vi "PWM Simulation.vi"() -> ()   [LabVIEW 2019]
uses:
  <vilib>/Simulation/Scripting/Companion Diagram/SimConfigNode/SimParams.ctl
  <vilib>/Simulation/Scripting/Companion Diagram/SimConfigNode/_simSolvers.ctl
  <vilib>/Simulation/Implementation/Shared/SIMSCR Execution Mode.ctl
  <vilib>/Platform/TimedLoop/XDataNode/timing_clust.ctl
  <vilib>/Platform/TimedLoop/XDataNode/nitl_modes.ctl
  <vilib>/Platform/TimedLoop/XDataNode/wakeup.ctl
  <vilib>/Simulation/Param Hierarchy/Typedefs/SIMPH Param Control Actions.ctl
  <vilib>/Simulation/Implementation/Shared/NILVSim_ParamChanged.vi
  <vilib>/Simulation/Implementation/Shared/NILVSim_FinishedLate.vi
  <vilib>/Simulation/Implementation/Shared/NILVSIM_BeginStep.vi
  <vilib>/Simulation/SignalDisplay/Implementation/NILVSim Time Waveform.llb/SIM Time Waveform (scalar).vi
  <vilib>/Simulation/Utility/Implementation/SIM Halt.vi
  <vilib>/Simulation/Implementation/Shared/NILVSim_Manager.vi
  <vilib>/Utility/error.llb/Clear Errors.vi
  <vilib>/Simulation/Implementation/Shared/NILVSim_FinalizeModel.vi
  <vilib>/Simulation/Implementation/Shared/SIM Unbundle Sim Info.vi
  <vilib>/Simulation/Implementation/Shared/SIMSH Read Queue.vi
  <vilib>/Simulation/Implementation/Shared/NILVSim_Initialize.vi
  Pulse Generator.vi
  <vilib>/Simulation/Utility/Implementation/NILVSim Get Time and IsAcceptedStep.vi
  <vilib>/Simulation/Implementation/Shared/NILVSim_GetModelError.vi
  <vilib>/Simulation/Implementation/Shared/SIM Bundle Sim Info.vi
  <vilib>/Simulation/Scripting/Companion Diagram/SimConfigNode/SimDog.xnode
  <vilib>/Platform/TimedLoop/XDataNode/XDataNode.xnode
  <vilib>/Simulation/Implementation/XNodeFramework/SimXNode/SimX.xnode
  <vilib>/Platform/TimedLoop/XDataNode/XDNodeRunTimeDep.lvlib
  <vilib>/Simulation/Implementation/Shared/NI_SIM_Implementation.lvlib
panel:
  in  "Stop Button":bool
  out "Threshold":dbl=50.0
  in  "Frequency (Hz)":dbl=1.0 min=0.0 max=10.0 step=0.01
  out "Boolean Pulse":waveform(dbl)(graph)={"t0"=timestamp(12.82 s since 1904-01-01), "dt"=1.0, "Y"=[0.0]}
  in  "Duty Cycle (%)":dbl(knob)=50.0 min=0.0 max=100.0 step=5.0 scale=0.0..100.0
  in  "Step size":dbl=0.01
  out "Counter":waveform(dbl)(graph)={"t0"=timestamp(12.82 s since 1904-01-01), "dt"=1.0, "Y"=[84.0]}
  out "Max Count":dbl=100.0
  # "Mechatronic Systems Board"
  # "Mechatronic Systems Board"
  # "PWM Simulation"
  # "Blob Detection"
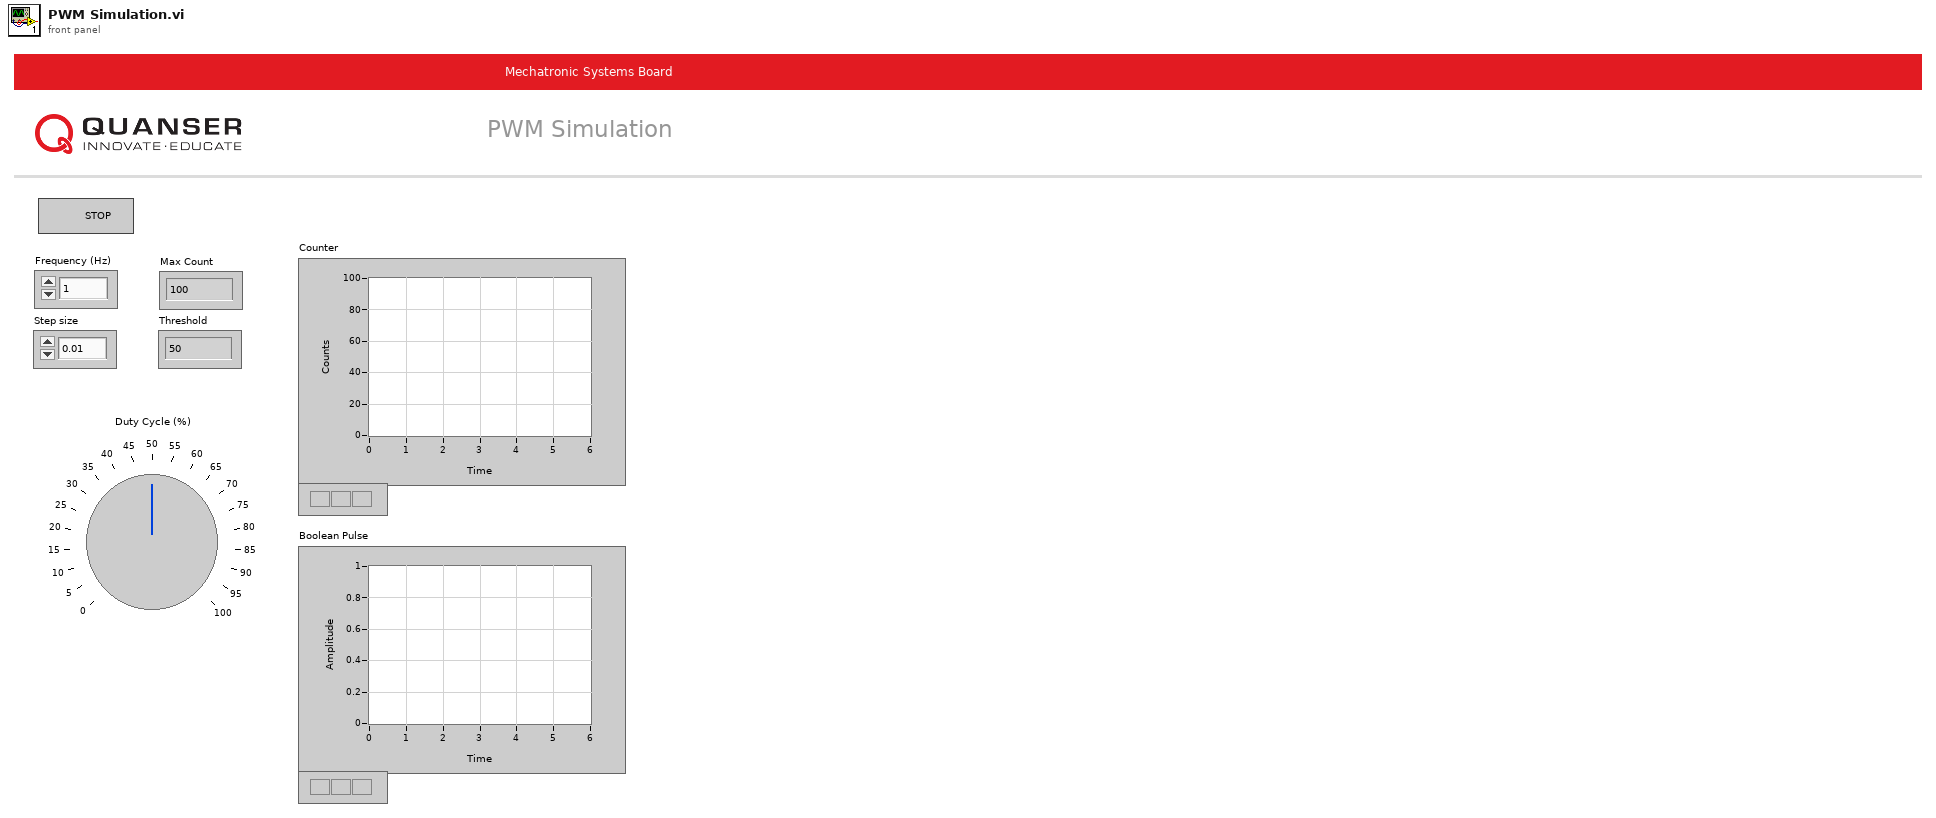
[diagram p1: front panel]
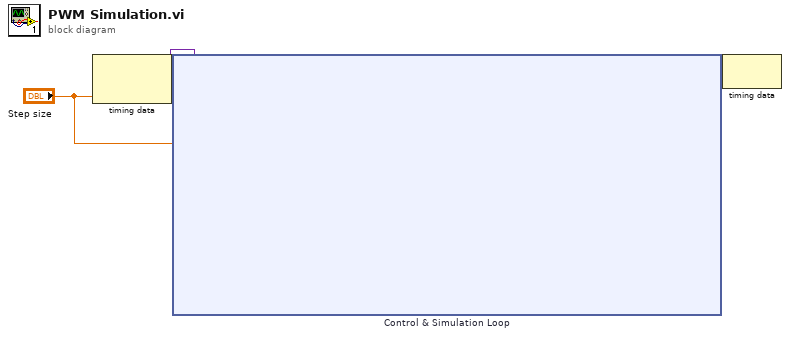
[diagram p0: block diagram]
diagram:
  n1 = node-c288("Step size") -> (w3:variant)  [unwired: 1 in]
  n2 = node-c254 "Control & Simulation Loop"(w3, "Step size") -> (w2:variant)
  n3 = node-c288(w2) -> ()  [unwired: 1 out]
